vi "Set Vertical Scale.vi"(8 "error in (no error)":errorcluster, 10 "Channels V/div":T1, 11 "VISA resource name":refnum<visa-resource-name>) -> (0 "error out":errorcluster, 3 "VISA resource name out":refnum<visa-resource-name>)   [LabVIEW 2018, in "DPO4104.lvlib" / "DPO4104.lvclass"]
doc: "This VI sends the command to set the volts per division."
uses:
  DPO4104.lvclass
  PPLs/Oscilloscope/Parent/Oscilloscope.lvlibp/Custom Controls/Volts per Division.ctl
  PPLs/Oscilloscope/Parent/Oscilloscope.lvlibp/Custom Controls/Analog Channels.ctl
  <instrlib>/Tektronix DPO MSO 2000 4000 Series/Tektronix DPO MSO 2000 4000 Series.lvlib
  PPLs/Oscilloscope/Parent/Oscilloscope.lvlibp
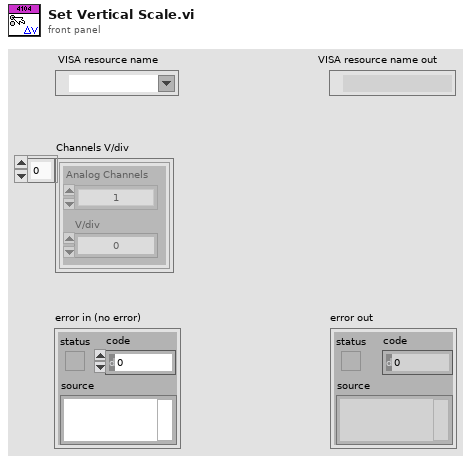
[diagram p1: front panel]
types:
  T1 = typedef "Oscilloscope.lvlibp/Volts per Division.ctl" = cluster{"Analog Channels":T2, "V/div":dbl}[]
  T2 = typedef "Oscilloscope.lvlibp/Analog Channels.ctl" = enum16{"1", "2", "3", "4", "5", "6", "7", "8", "9", "10", "11", "12", "13", "14", "15", "16"}
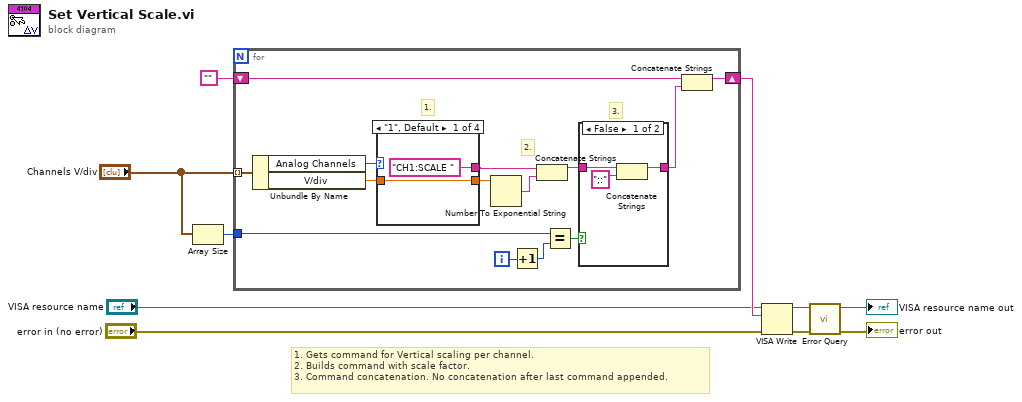
[diagram p0: block diagram]
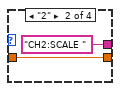
[diagram p3: hidden frame]
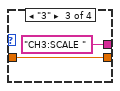
[diagram p4: hidden frame]
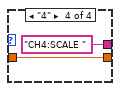
[diagram p5: hidden frame]
diagram:
  # "1. Gets command for Vertical scaling per channel.\n2. Builds command with scale factor.\n3. Command concatenation. No concatenation after last command appended."
  n1 = Array Size(array="Channels V/div") -> (size(s)=w1:i32)
  n2 = for {
    tunnel: "Channels V/div" -> [w24] mode=indexing
    shift-right: [w17] -> w5
    shift-left: "" -> [w16]
    tunnel: w1 -> [w19]
    i -> [w21]
    # "2."
    # "3."
    # "1."
    n3 = Unbundle By Name(w24) -> ("Analog Channels"=w23:T2, "V/div"=w22:dbl)
    n4 = case shown="\"1\", Default" w23 {
      tunnel: w22 -> [w29 w31 w33 w35]
      tunnel: ["CH1:SCALE " "CH2:SCALE " "CH3:SCALE " "CH4:SCALE "] -> w13
      tunnel: [w29 w31 w33 w35] -> w12
      frame "1", Default {
      }
      frame "2" {
      }
      frame "3" {
      }
      frame "4" {
      }
    }
    n5 = Number To Exponential String(number=w12) -> (E-format string=w14:string)  [unwired: 3 in]
    n6 = Increment(x=w21) -> (x+1=w20:i32)
    n7 = Concatenate Strings(w13, w14) -> (w11:string)
    n8 = Equal?(x=w19, y=w20) -> (x = y?=w18:bool)
    n9 = case shown="False" w18 {
      tunnel: w11 -> [w27 w28]
      tunnel: [w25 w28] -> w15
      frame False {
        n10 = Concatenate Strings(w27, ";:" ("string")) -> (w25:string)
      }
      frame True {
      }
    }
    n11 = Concatenate Strings(w16, w15) -> (w17:string)
  }
  n12 = VISA Write(VISA resource name="VISA resource name", write buffer=w5, error in (no error)="error in (no error)") -> (VISA resource name out=w10:refnum<visa-resource-name>, error out=w9:errorcluster)  [unwired: 1 out]
  n13 = call <instrlib>:"Error Query.vi"("error in (no error)"=w9, "VISA resource name"=w10) -> ("error out"=→"error out":errorcluster, "VISA resource name out"=→"VISA resource name out":refnum<visa-resource-name>)  [unwired: 6 in, 2 out]
